vi "rename channel.vi"(8 "error in":errorcluster, 9 "new name":string, 10 "old name":string, 11 "TDMS datalogger configuration in":refnum<class "TDMS datalogger configuration.lvclass">) -> (0 "error out":errorcluster, 3 "TDMS datalogger configuration out":refnum<class "TDMS datalogger configuration.lvclass">)   [LabVIEW 2013, in "TDMS datalogger configuration.lvclass"]
uses:
  TDMS datalogger configuration.lvclass
  TDMS datalogger configuration.lvclass/TDMS datalogger configuration.ctl
  <vilib>/NI/Tag Bus/tag/tag descriptor.lvclass/tag descriptor.ctl
  <vilib>/NI/Tag Bus/tag/read tag name.vi
  <vilib>/NI/Tag Bus/tag/tag descriptor.lvclass
  <vilib>/NI/Tag Bus Module Framework/root configuration/TBM configuration.lvclass
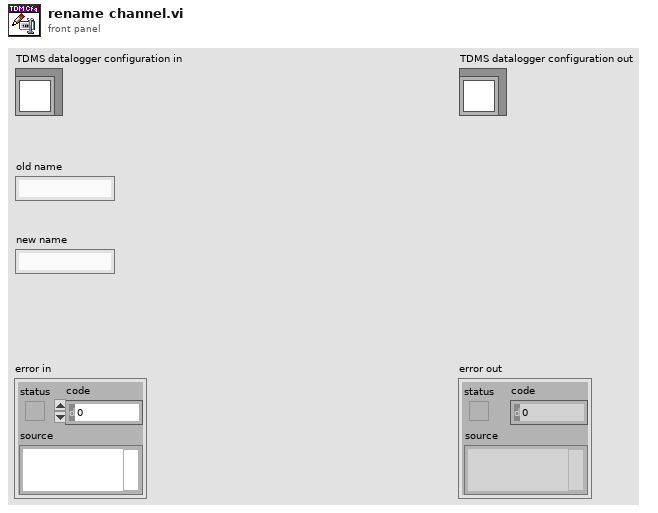
[diagram p1: front panel]
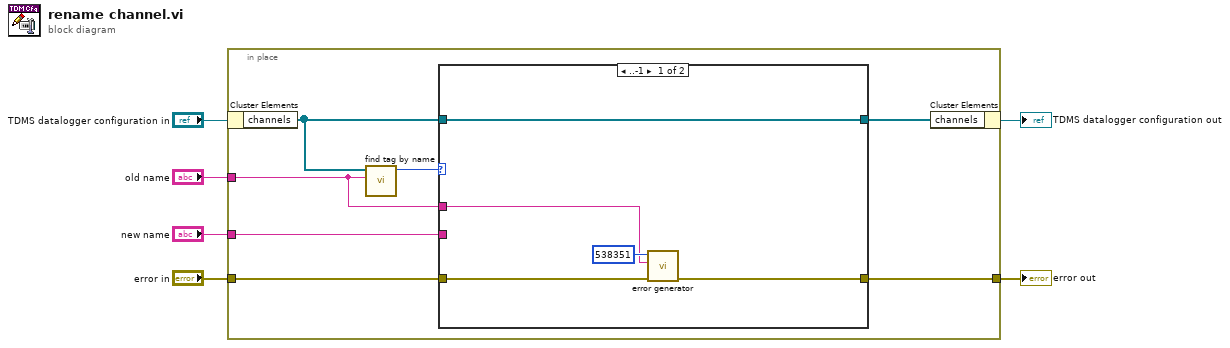
[diagram p0: block diagram]
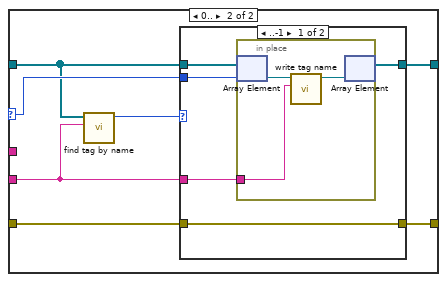
[diagram p2: hidden frame]
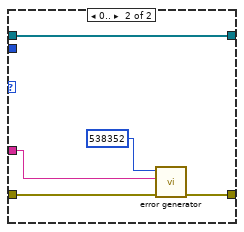
[diagram p3: hidden frame]
diagram:
  n1 = in-place {
    in-place-border: "old name" -> [w8]
    in-place-border: "new name" -> [w10]
    in-place-border: [w13] -> w1
    in-place-border: "error in" -> [w11]
    n2 = in-place-cluster #1("TDMS datalogger configuration in") -> ("channels"=w9:refnum<class "TBM channel.lvclass">[])
    n3 = call <vilib>:"find tag by name.vi"("name"=w8, "tags in"=w9) -> ("index"=w7:i32)  [unwired: 9 in]
    n4 = case shown="..-1" w7 {
      selector: w7 -> [_ w22]
      tunnel: w9 -> [w15 w21]
      tunnel: w8 -> [w17 _]
      tunnel: [w16 w23] -> w13
      tunnel: [w15 w25] -> w12
      tunnel: w11 -> [w14 w24]
      tunnel: w10 -> [_ w20]
      frame ..-1 {
        n5 = call <vilib>:"error generator.vi"("error in"=w14, "append error message"=w17, "error code (0)"=538351) -> ("error out"=w16:errorcluster)  [unwired: 8 in]
      }
      frame 0.. {
        n6 = call <vilib>:"find tag by name.vi"("name"=w20, "tags in"=w21) -> ("index"=w19:i32)  [unwired: 9 in]
        n7 = case shown="..-1" w19 {
          tunnel: [w30 w38] -> w25
          tunnel: w22 -> [w29 _]
          tunnel: w21 -> [w28 w38]
          tunnel: w20 -> [w27 w34]
          tunnel: w24 -> [w26 w36]
          tunnel: [w26 w37] -> w23
          frame ..-1 {
            n8 = in-place {
              in-place-border: w27 -> [w31]
              n9 = in-place-array #2(w28, w29) -> (w33:refnum<class "TBM channel.lvclass">)
              n10 = call <vilib>:"write tag name.vi"("name"=w31, "system tag in"=w33) -> ("system tag out"=w32:refnum<class "TBM channel.lvclass">)  [unwired: 8 in, 1 out]
              n11 = in-place-array #2(w32) -> (w30:refnum<class "TBM channel.lvclass">[])  [unwired: 1 out]
            }
          }
          frame 0.. {
            n12 = call <vilib>:"error generator.vi"("error in"=w36, "append error message"=w34, "error code (0)"=538352) -> ("error out"=w37:errorcluster)  [unwired: 8 in]
          }
        }
      }
    }
    n13 = in-place-cluster #1("channels"=w12) -> (→"TDMS datalogger configuration out":refnum<class "TDMS datalogger configuration.lvclass">)
  }
  "error out" <- w1
